vi "Test Helper VI Error Handling when Logger Not Initialized.vi"(8 "error in":errorcluster) -> (0 "error out":errorcluster)   [LabVIEW 2016, in "UT_Helper.lvlib"]
doc: "Test if there is no error after an existent Logger was closed.\nTest if there is an error after the close was called again."
uses:
  UT_Helper.lvlib
  <vilib>/Utility/error.llb/Error Cluster From Error Code.vi
  <vilib>/ErrorRing/Error Ring.xnode
  <vilib>/addons/_JKI Toolkits/Caraya/classes/Test/Test.lvclass
  Source/HSE-Logger/hse-logger.lvlib
  <vilib>/addons/_JKI Toolkits/Caraya/classes/Assert/Assert.lvclass
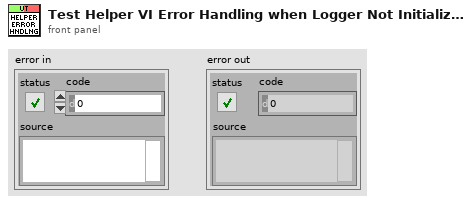
[diagram p1: front panel]
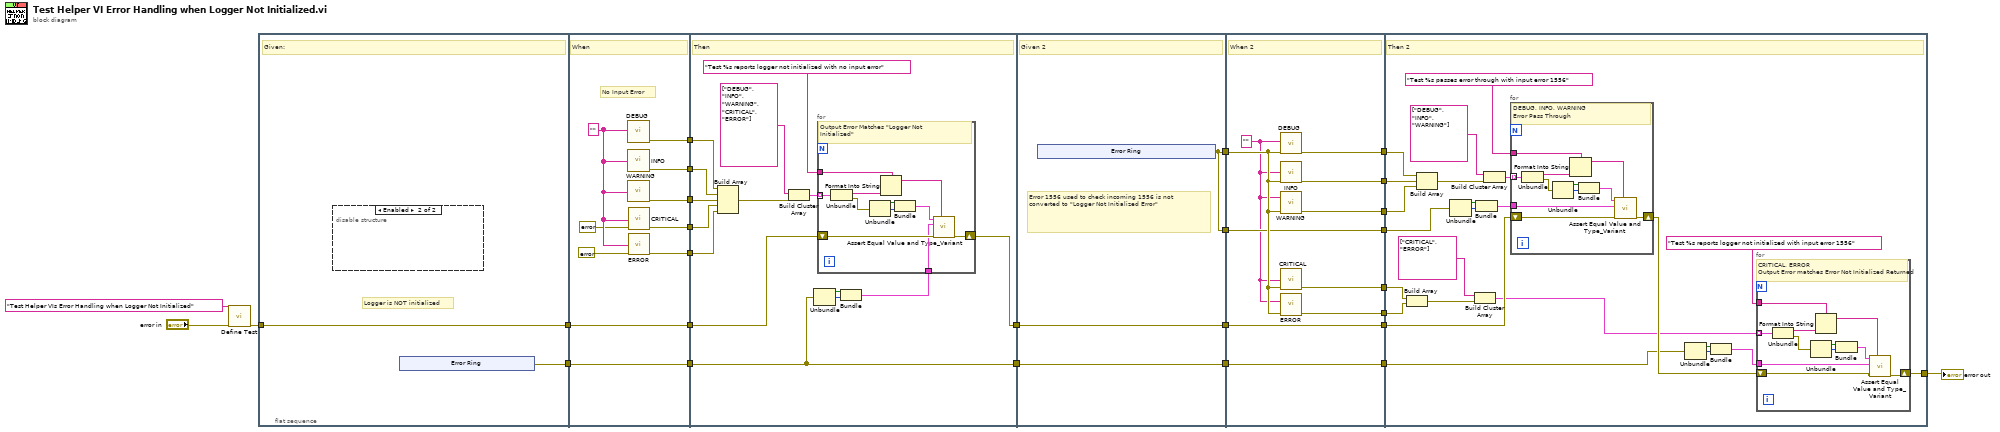
[diagram p0: block diagram]
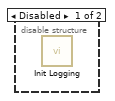
[diagram p2: hidden frame]
diagram:
  n1 = call <vilib>:"Define Test.vi"("error in (no error)"="error in", "Label (VI Title)"="Test Helper VIs Error Handling when Logger Not Initialized") -> ("error out"=w26:errorcluster)  [unwired: 8 in, 1 out]
  n2 = flat-sequence {
    tunnel: w26 -> [w29]
    tunnel: [w29] -> w18
    tunnel: [w28] -> w3
    tunnel: w18 -> [w40]
    tunnel: [w40] -> w16
    tunnel: [w39] -> w15
    tunnel: [w38] -> w14
    tunnel: [w37] -> w13
    tunnel: [w36] -> w12
    tunnel: [w35] -> w11
    tunnel: [w34] -> w4
    tunnel: w3 -> [w34]
    tunnel: w16 -> [w50]
    tunnel: w15 -> [w55]
    tunnel: w14 -> [w54]
    tunnel: w13 -> [w53]
    tunnel: w12 -> [w52]
    tunnel: w11 -> [w51]
    tunnel: [w49] -> w10
    tunnel: [w48] -> w7
    tunnel: w4 -> [w48]
    tunnel: [w69] -> w19
    tunnel: [w67] -> w17
    tunnel: w10 -> [w69]
    tunnel: [w68] -> w8
    tunnel: w7 -> [w68]
    tunnel: [w67] -> w6
    tunnel: [w83] -> w25
    tunnel: [w82] -> w24
    tunnel: [w81] -> w23
    tunnel: [w80] -> w22
    tunnel: [w79] -> w21
    tunnel: [w78] -> w20
    tunnel: w19 -> [w78]
    tunnel: w17 -> [w77]
    tunnel: [w76] -> w9
    tunnel: w8 -> [w76]
    tunnel: w6 -> [w75]
    tunnel: [w75] -> w5
    tunnel: w25 -> [w107]
    tunnel: w24 -> [w106]
    tunnel: w23 -> [w105]
    tunnel: w22 -> [w104]
    tunnel: w21 -> [w103]
    tunnel: [w101] -> w2
    tunnel: w20 -> [w100]
    tunnel: w9 -> [w98]
    tunnel: w5 -> [w99]
    frame #0 {
      # "Logger is NOT initialized"
      # "Given:"
      n3 = disable-structure "Diagram Disable Structure" shown="Enabled" {
        frame Disabled {
          n4 = call "Init Logging.vi"() -> ()  [unwired: 11 in, 1 out]
        }
        frame Enabled {
        }
      }
      n5 = xnode ("Error Ring")() -> ("error out"=w28:errorcluster)
    }
    frame #1 {
      w33 = "" ("Message")
      # "No Input Error"
      # "When"
      n6 = call "DEBUG.vi"("Message"=w33) -> ("error out"=w39:errorcluster)  [unwired: 10 in]
      n7 = call "INFO.vi"("Message"=w33) -> ("error out"=w38:errorcluster)  [unwired: 10 in]
      n8 = call "WARNING.vi"("Message"=w33) -> ("error out"=w37:errorcluster)  [unwired: 10 in]
      n9 = call "CRITICAL.vi"("Message"=w33, "error in"=errorcluster {"status"=FALSE, "code"=0, "source"=""}) -> ("error out"=w36:errorcluster)  [unwired: 9 in]
      n10 = call "ERROR.vi"("Message"=w33, "error in"=errorcluster {"status"=FALSE, "code"=0, "source"=""}) -> ("error out"=w35:errorcluster)  [unwired: 9 in]
    }
    frame #2 {
      # "Then"
      n11 = Build Array(w55, w54, w53, w52, w51) -> (w47:errorcluster[])
      n12 = Build Cluster Array ("Index & Bundle Cluster Array")(string[] ["DEBUG", "INFO", "WARNING", "CRITICAL", "ERROR"], w47) -> (w45:cluster{string, "error out":errorcluster}[])
      n13 = Unbundle(w48) -> ("status"=w41:bool, "code"=w42:i32)  [unwired: 1 out]
      n14 = Bundle("status"=w41, "code"=w42) -> (w43:cluster{"status":bool, "code":i32})  [unwired: 1 in]
      n15 = for {
        tunnel: w45 -> [w63] mode=indexing
        shift-right: [w65] -> w49
        shift-left: w50 -> [w66]
        tunnel: "Test %s reports logger not initialized with no input error" ("format string") -> [w60]
        tunnel: w43 -> [w59]
        # "Output Error Matches \"Logger Not Initialized\""
        n16 = Unbundle(w63) -> (w62:string, "error out"=w64:errorcluster)
        n17 = Unbundle(w64) -> ("status"=w58:bool, "code"=w57:i32)  [unwired: 1 out]
        n18 = Format Into String(format string=w60, w62) -> (resulting string=w61:string)  [unwired: 2 in, 1 out]
        n19 = Bundle("status"=w58, "code"=w57) -> (w56:cluster{"status":bool, "code":i32})  [unwired: 1 in]
        n20 = call <vilib>:"Assert Equal Value and Type_Variant.vi"("Label"=w61, "error in (no error)"=w66, "Y"=w59, "X"=w56) -> ("error out"=w65:errorcluster)  [unwired: 6 in, 1 out]
      }
    }
    frame #3 {
      # "Error 1556 used to check incoming 1556 is not converted to \"Logger Not Initialized Error\""
      # "Given 2"
      n21 = xnode ("Error Ring")() -> ("error out"=w67:errorcluster)
    }
    frame #4 {
      w74 = "" ("Message")
      # "When 2"
      n22 = call "DEBUG.vi"("Message"=w74, "error in"=w77) -> ("error out"=w83:errorcluster)  [unwired: 9 in]
      n23 = call "INFO.vi"("Message"=w74, "error in"=w77) -> ("error out"=w82:errorcluster)  [unwired: 9 in]
      n24 = call "WARNING.vi"("Message"=w74, "error in"=w77) -> ("error out"=w81:errorcluster)  [unwired: 9 in]
      n25 = call "CRITICAL.vi"("Message"=w74, "error in"=w77) -> ("error out"=w80:errorcluster)  [unwired: 9 in]
      n26 = call "ERROR.vi"("Message"=w74, "error in"=w77) -> ("error out"=w79:errorcluster)  [unwired: 9 in]
    }
    frame #5 {
      # "Then 2"
      n27 = Build Array(w104, w103) -> (w94:errorcluster[])
      n28 = Build Array(w107, w106, w105) -> (w97:errorcluster[])
      n29 = Unbundle(w99) -> ("status"=w89:bool, "code"=w88:i32)  [unwired: 1 out]
      n30 = Build Cluster Array ("Index & Bundle Cluster Array")(string[] ["CRITICAL", "ERROR"], w94) -> (w92:cluster{string, "error out":errorcluster}[])
      n31 = Bundle("status"=w89, "code"=w88) -> (w87:cluster{"status":bool, "code":i32})  [unwired: 1 in]
      n32 = Build Cluster Array ("Index & Bundle Cluster Array")(string[] ["DEBUG", "INFO", "WARNING"], w97) -> (w95:cluster{string, "error out":errorcluster}[])
      n33 = for {
        tunnel: w95 -> [w126] mode=indexing
        shift-right: [w128] -> w102
        shift-left: w100 -> [w129]
        tunnel: "Test %s passes error through with input error 1556" ("format string") -> [w123]
        tunnel: w87 -> [w119]
        # "DEBUG, INFO, WARNING \nError Pass Through"
        n34 = Unbundle(w126) -> (w125:string, "error out"=w127:errorcluster)
        n35 = Unbundle(w127) -> ("status"=w121:bool, "code"=w122:i32)  [unwired: 1 out]
        n36 = Format Into String(format string=w123, w125) -> (resulting string=w124:string)  [unwired: 2 in, 1 out]
        n37 = Bundle("status"=w121, "code"=w122) -> (w120:cluster{"status":bool, "code":i32})  [unwired: 1 in]
        n38 = call <vilib>:"Assert Equal Value and Type_Variant.vi"("Label"=w124, "error in (no error)"=w129, "Y"=w119, "X"=w120) -> ("error out"=w128:errorcluster)  [unwired: 6 in, 1 out]
      }
      n39 = Unbundle(w98) -> ("status"=w86:bool, "code"=w85:i32)  [unwired: 1 out]
      n40 = Bundle("status"=w86, "code"=w85) -> (w84:cluster{"status":bool, "code":i32})  [unwired: 1 in]
      n41 = for {
        shift-right: [w118] -> w101
        shift-left: w102 -> [w117]
        tunnel: w92 -> [w114] mode=indexing
        tunnel: "Test %s reports logger not initialized with input error 1556" ("format string") -> [w113]
        tunnel: w84 -> [w111]
        # "CRITICAL, ERROR\nOutput Error matches Error Not Initialized Returned"
        n42 = Unbundle(w114) -> (w115:string, "error out"=w116:errorcluster)
        n43 = Unbundle(w116) -> ("status"=w110:bool, "code"=w109:i32)  [unwired: 1 out]
        n44 = Format Into String(format string=w113, w115) -> (resulting string=w112:string)  [unwired: 2 in, 1 out]
        n45 = Bundle("status"=w110, "code"=w109) -> (w108:cluster{"status":bool, "code":i32})  [unwired: 1 in]
        n46 = call <vilib>:"Assert Equal Value and Type_Variant.vi"("Label"=w112, "error in (no error)"=w117, "Y"=w111, "X"=w108) -> ("error out"=w118:errorcluster)  [unwired: 6 in, 1 out]
      }
    }
  }
  "error out" <- w2
